vi "proc_demo.vi"() -> ()   [LabVIEW 2012]
panel:
  out "read buffer 2":string
  out "bytes written":i32
  out "exit code":i32
  out "bytes read":i32
  out "bytes to read":i32
  out "read buffer":string
  out "error out":errorcluster
  in  "command":string
  in  "folder":string
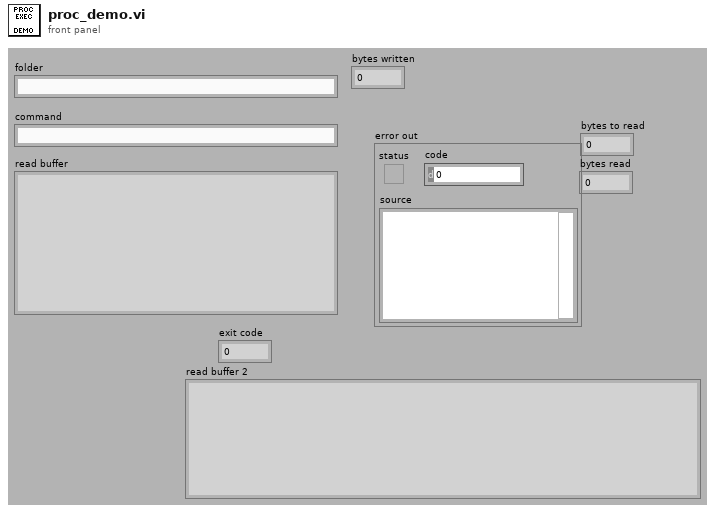
[diagram p1: front panel]
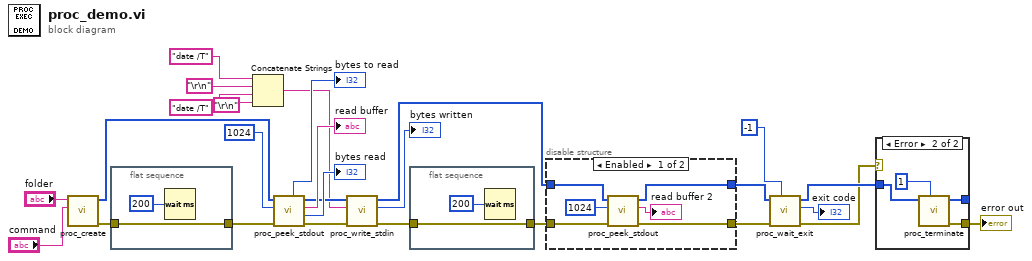
[diagram p0: block diagram]
diagram:
  n1 = call "proc_create.vi"("command"="command", "folder"="folder") -> ("error out"=w20:errorcluster, "process instance handle"=w26:u32[])  [unwired: 8 in]
  n2 = flat-sequence {
    tunnel: [w29] -> w19
    tunnel: w20 -> [w29]
    frame #0 {
      n3 = Wait (ms)(milliseconds to wait=u32 200) -> ()  [unwired: 1 out]
    }
  }
  n4 = Concatenate Strings("date /T" ("write buffer"), "\r\n", "date /T" ("write buffer"), "\r\n") -> (w12:string)
  n5 = call "proc_peek_stdout.vi"("error in"=w19, "size"=1024, "process instance handle in"=w26) -> ("error out"=w16:errorcluster, "bytes read"=→"bytes read":i32, "read buffer"=→"read buffer":string, "process instance handle out"=w15:u32[], "bytes to read"=→"bytes to read":i32)  [unwired: 3 in, 1 out]
  n6 = call "proc_write_stdin.vi"("error in"=w16, "write buffer"=w12, "process instance handle in"=w15) -> ("error out"=w11:errorcluster, "bytes written"=→"bytes written":i32, "process instance handle out"=w4:u32[])  [unwired: 6 in]
  n7 = flat-sequence {
    tunnel: [w30] -> w6
    tunnel: w11 -> [w30]
    frame #0 {
      n8 = Wait (ms)(milliseconds to wait=u32 200) -> ()  [unwired: 1 out]
    }
  }
  n9 = disable-structure shown="Enabled" {
    disable-tunnel: w6 -> [w37 w38]
    disable-tunnel: [w36 w38] -> w5
    disable-tunnel: w4 -> [w35 w39]
    disable-tunnel: [w34 w39] -> w3
    frame Enabled {
      n10 = call "proc_peek_stdout.vi"("error in"=w37, "size"=1024, "process instance handle in"=w35) -> ("error out"=w36:errorcluster, "read buffer"=→"read buffer 2":string, "process instance handle out"=w34:u32[])  [unwired: 3 in, 3 out]
    }
    frame Disabled {
    }
  }
  n11 = call "proc_wait_exit.vi"("timeout [ms]"=-1, "error in"=w5, "process instance handle in"=w3) -> ("error out"=w1:errorcluster, "exit code"=→"exit code":i32, "process instance handle out"=w17:u32[])  [unwired: 6 in]
  n12 = case shown="Error" w1 {
    selector: w1 -> [w40 _]
    tunnel: w17 -> [w41 w45]
    tunnel: [w40 w42] -> w9
    tunnel: [w41 w43] -> _
    frame No Error {
    }
    frame Error {
      n13 = call "proc_terminate.vi"("timeout [ms]"=1, "process instance handle in"=w45) -> ("error out"=w42:errorcluster, "process instance handle out"=w43:u32[])  [unwired: 8 in]
    }
  }
  "error out" <- w9
